vi "Single Input Impedance.vi"(8 "error in":errorcluster, 9 "Impedance":T1 items=["50 Ohm", "1M Ohm"], 10 "Channel":i32(ring) items=["Input Channel 1", "Input Channel 2", "Input Channel 3", "Input Channel 4"], 11 "Instrument Handle In":i32) -> (0 "error out":errorcluster, 3 "Instrument Handle Out":i32)   [LabVIEW 8.6, in "ZTScopeM.lvlib"]
doc: "Configure the input impedance for the selected channel."
uses:
  ZTScopeM.lvlib
  Impedance.ctl
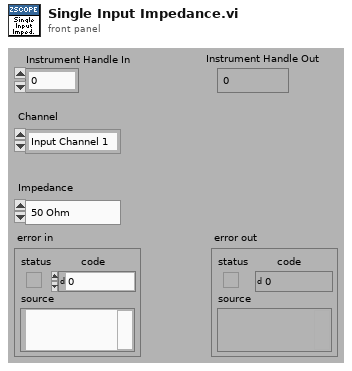
[diagram p1: front panel]
types:
  T1 = typedef "ZTScopeM.lvlib/Impedance.ctl" = dbl
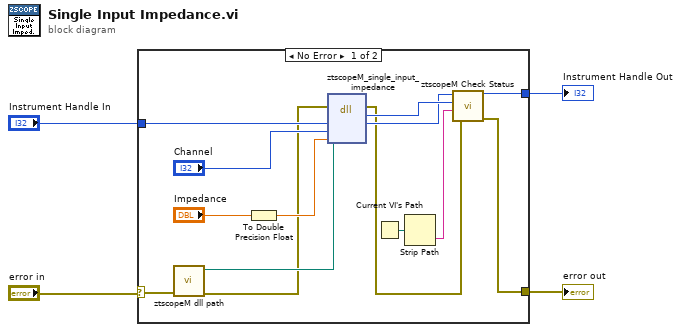
[diagram p0: block diagram]
diagram:
  n1 = case shown="No Error" "error in" {
    selector: "error in" -> [w9 w20]
    tunnel: [w13 w20] -> w3
    tunnel: [w14 w19] -> w2
    tunnel: "Instrument Handle In" -> [w7 w19]
    frame #0 {
      n2 = call "ztscopeM dll path.vi"("error in (no error)"=w9) -> ("error out"=w6:errorcluster, "<instrument>.dll path"=w8:path)  [unwired: 9 in]
      n3 = To Double Precision Float(number="Impedance") -> (double precision float=w10:T1)
      n4 = dll-call lib="C:/Program Files (x86)/National Instruments/LabVIEW 2013/instr.lib/ztscopem/ztscopeM.dll" fn="ztscopeM_single_input_impedance"(path in=w8, error in=w6, "instrumentHandle"=w7, "channel"="Channel", "impedance"=w10) -> (error out=w5:errorcluster, "return type"=w18:i32, "instrumentHandle"=w17:i32)  [unwired: 3 in, 1 out]
      n5 = Current VI's Path() -> (path=w16:path)
      n6 = Strip Path(path=w16) -> (name=w15:string)  [unwired: 1 out]
      n7 = call "ztscopeM Check Status.vi"("error in"=w5, "name of VI"=w15, "status (return code)"=w18, "instrument handle in"=w17) -> ("error out"=w13:errorcluster, "instrument handle out"=w14:i32)  [unwired: 2 out]
    }
    frame #1 {
    }
  }
  "Instrument Handle Out" <- w2
  "error out" <- w3
